vi "Write status.vi"(6 "hold if empty":bool, 8 "error in (no error)":errorcluster, 10 "status":T1, 11 "Motor in":refnum<class "Motor.lvclass">) -> (0 "error out":errorcluster, 3 "Motor out":refnum<class "Motor.lvclass">)   [LabVIEW 2018, in "Motor.lvclass"]
uses:
  Motor.lvclass
  Motor.lvclass/Motor.ctl
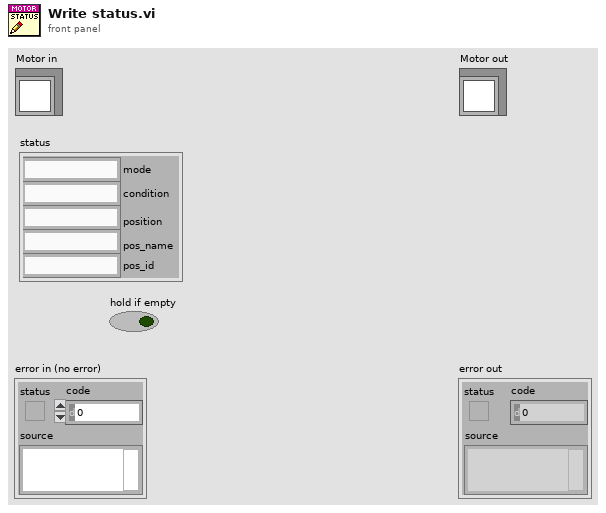
[diagram p1: front panel]
types:
  T1 = cluster{"mode":string, "condition":string, "position":string, "pos_name":string, "pos_id":string}
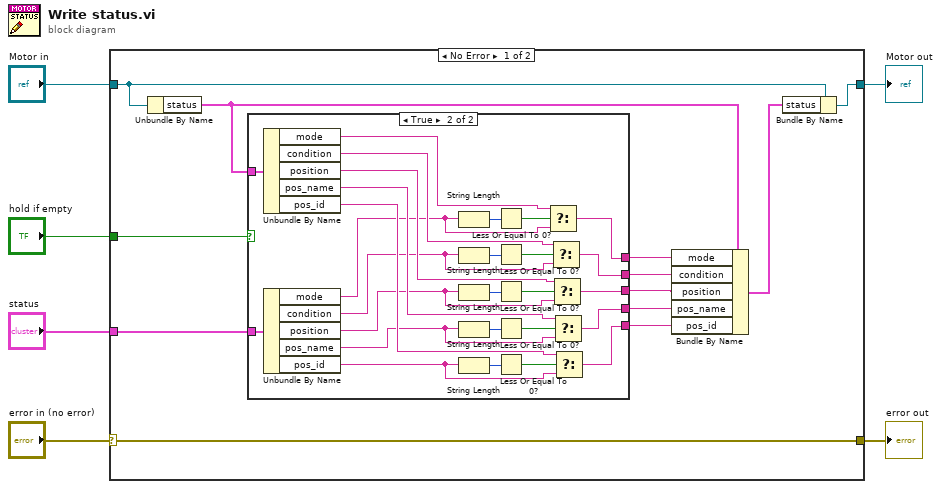
[diagram p0: block diagram]
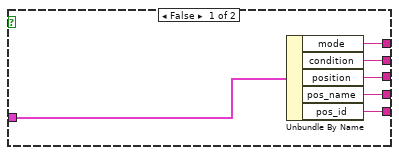
[diagram p2: hidden frame]
diagram:
  n1 = case shown="No Error" "error in (no error)" {
    selector: "error in (no error)" -> [w18 w52]
    tunnel: [w18 w52] -> w5
    tunnel: [w17 w53] -> w3
    tunnel: "Motor in" -> [w14 w53]
    tunnel: "status" -> [w13 _]
    tunnel: "hold if empty" -> [w12 _]
    frame No Error {
      n2 = Unbundle By Name(w14) -> ("status"=w16:T1)
      n3 = case shown="True" w12 {
        tunnel: w16 -> [_ w51]
        tunnel: w13 -> [w19 w50]
        tunnel: [w24 w27] -> w11
        tunnel: [w23 w26] -> w10
        tunnel: [w21 w46] -> w9
        tunnel: [w20 w43] -> w8
        tunnel: [w22 w25] -> w7
        frame False {
          n4 = Unbundle By Name(w19) -> ("mode"=w24:string, "condition"=w23:string, "position"=w22:string, "pos_name"=w21:string, "pos_id"=w20:string)
        }
        frame True {
          n5 = Unbundle By Name(w51) -> ("mode"=w34:string, "condition"=w33:string, "position"=w32:string, "pos_name"=w47:string, "pos_id"=w41:string)
          n6 = Unbundle By Name(w50) -> ("mode"=w31:string, "condition"=w30:string, "position"=w29:string, "pos_name"=w28:string, "pos_id"=w42:string)
          n7 = String Length(string=w31) -> (length=w35:i32)
          n8 = String Length(string=w30) -> (length=w38:i32)
          n9 = String Length(string=w29) -> (length=w39:i32)
          n10 = String Length(string=w28) -> (length=w49:i32)
          n11 = String Length(string=w42) -> (length=w44:i32)
          n12 = Less Or Equal To 0?(x=w35) -> (x <= 0?=w36:bool)
          n13 = Less Or Equal To 0?(x=w38) -> (x <= 0?=w37:bool)
          n14 = Less Or Equal To 0?(x=w39) -> (x <= 0?=w40:bool)
          n15 = Less Or Equal To 0?(x=w49) -> (x <= 0?=w48:bool)
          n16 = Less Or Equal To 0?(x=w44) -> (x <= 0?=w45:bool)
          n17 = Select(t=w34, s=w36, f=w31) -> (s? t:f=w27:string)
          n18 = Select(t=w33, s=w37, f=w30) -> (s? t:f=w26:string)
          n19 = Select(t=w32, s=w40, f=w29) -> (s? t:f=w25:string)
          n20 = Select(t=w47, s=w48, f=w28) -> (s? t:f=w46:string)
          n21 = Select(t=w41, s=w45, f=w42) -> (s? t:f=w43:string)
        }
      }
      n22 = Bundle By Name(cluster=w16, "mode"=w11, "condition"=w10, "position"=w7, "pos_name"=w9, "pos_id"=w8) -> (w15:T1)
      n23 = Bundle By Name(cluster=w14, "status"=w15) -> (w17:refnum<class "Motor.lvclass">)
    }
    frame Error {
    }
  }
  "error out" <- w5
  "Motor out" <- w3
